vi "Get_data.vi"() -> (0 "EOF? and Error status":bool, 6 "Block Header":string)   [LabVIEW 2022 SP3]
uses:
  Controls/Block_start_and_end.ctl
  Controls/Trigger_Mode.ctl
  Globals/Meas_global.vi
  Globals/Preference_global.vi
  Globals/Trav_pos_global.vi
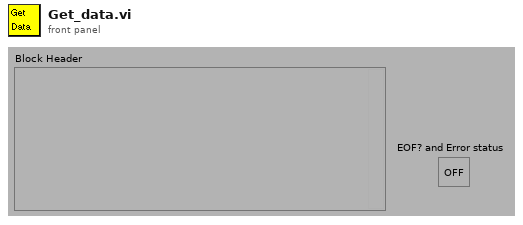
[diagram p1: front panel]
types:
  T1 = typedef "Block_start_and_end.ctl" = cluster{"Started":dbl, "Ended":dbl}
  T2 = typedef "Trigger_Mode.ctl" = enum16{"Free Running", "Start on Trigger", "Trigger Every Block", "Trigger Every Sample"}
  T3 = typedef "Post_Process.ctl" = enum16{"Take New Data", "Post Process Raw Data File"}
  T4 = typedef "PWA_Data.ctl" = enum16{"No PWA Data", "One Ch PWA"}
  T5 = typedef "Rendezvous RefNum" = refnum<k1>
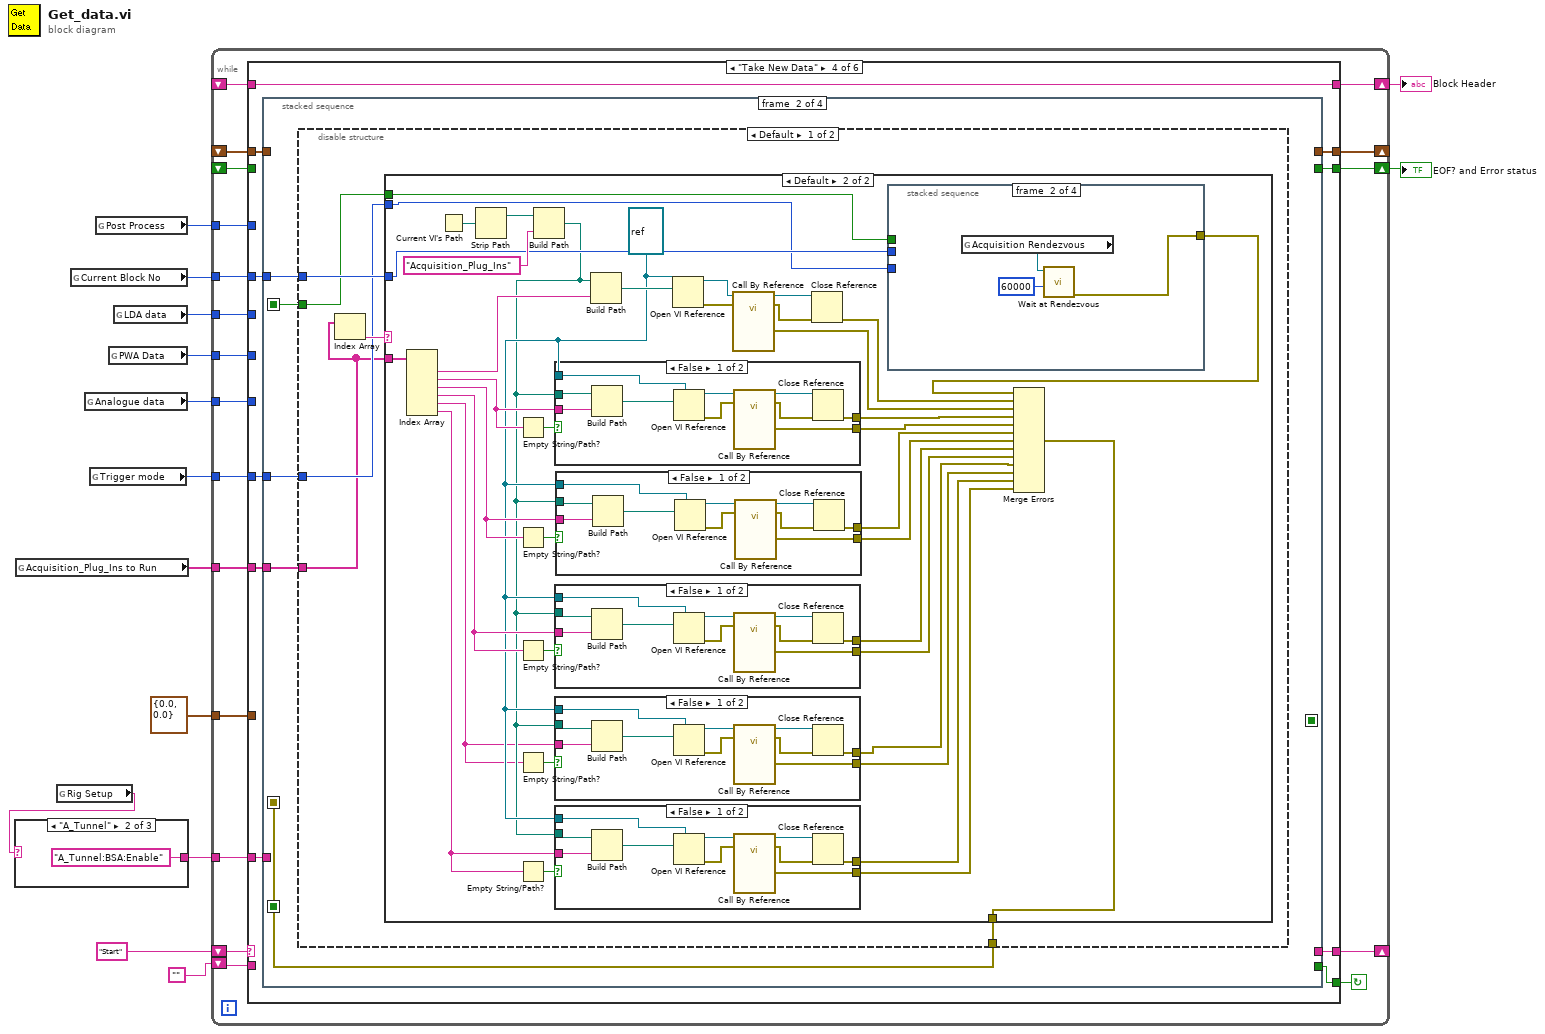
[diagram p0: block diagram]
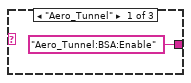
[diagram p2: hidden frame]
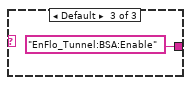
[diagram p3: hidden frame]
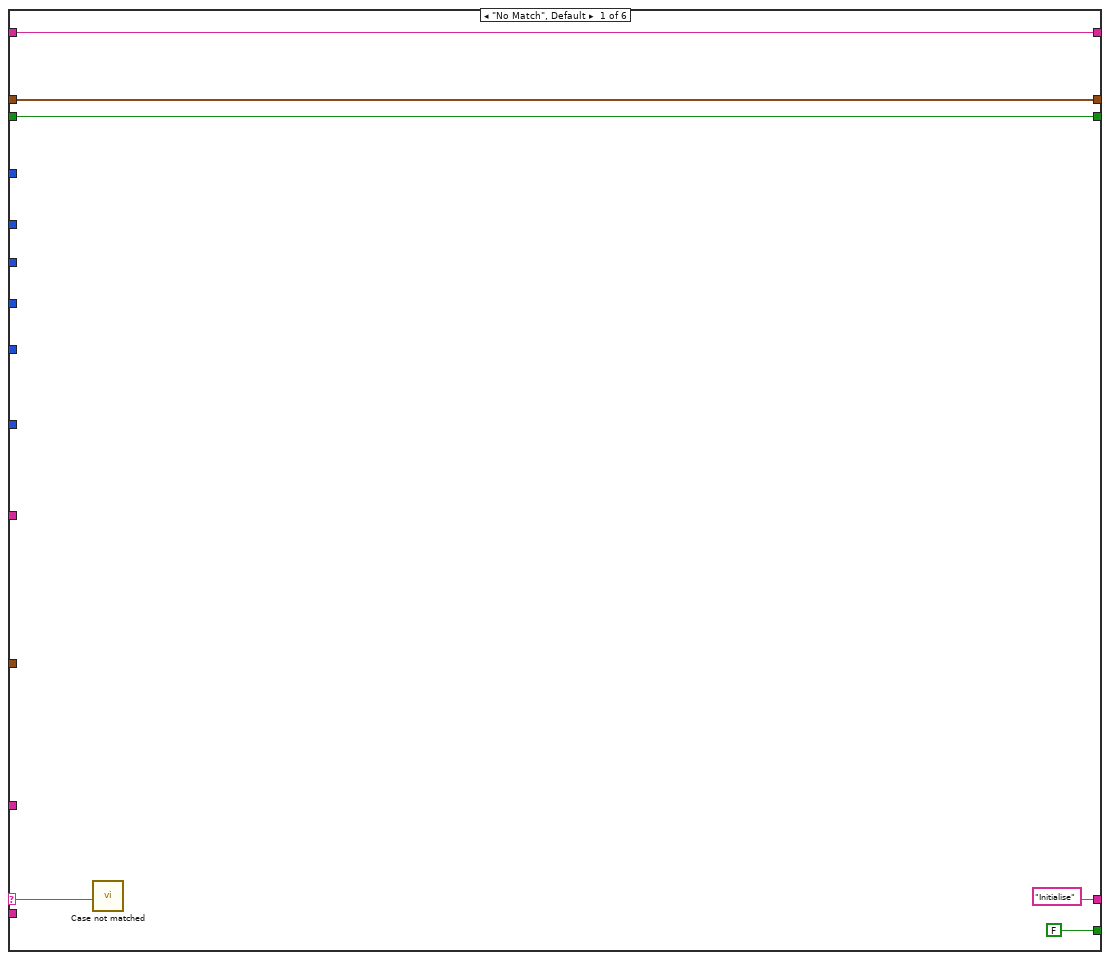
[diagram p4: hidden frame]
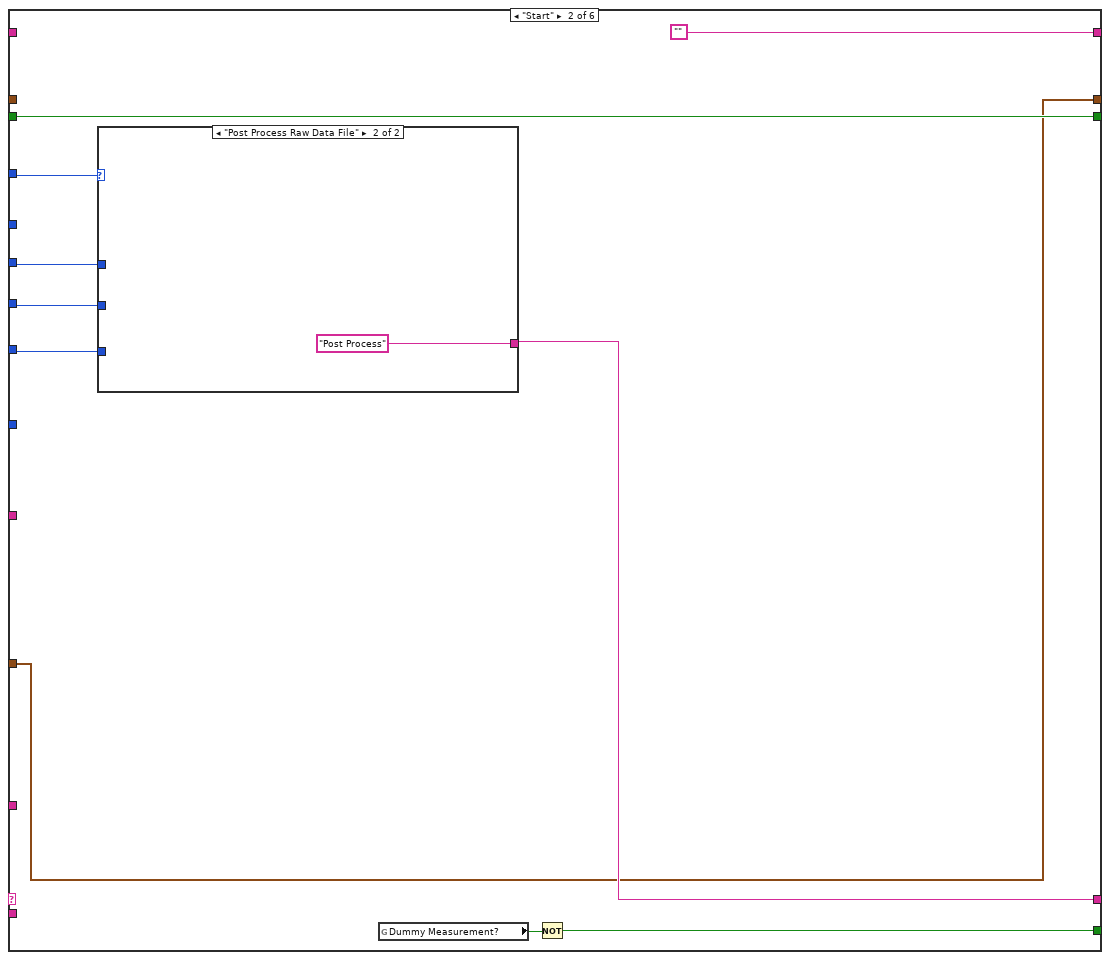
[diagram p5: hidden frame]
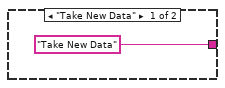
[diagram p6: hidden frame]
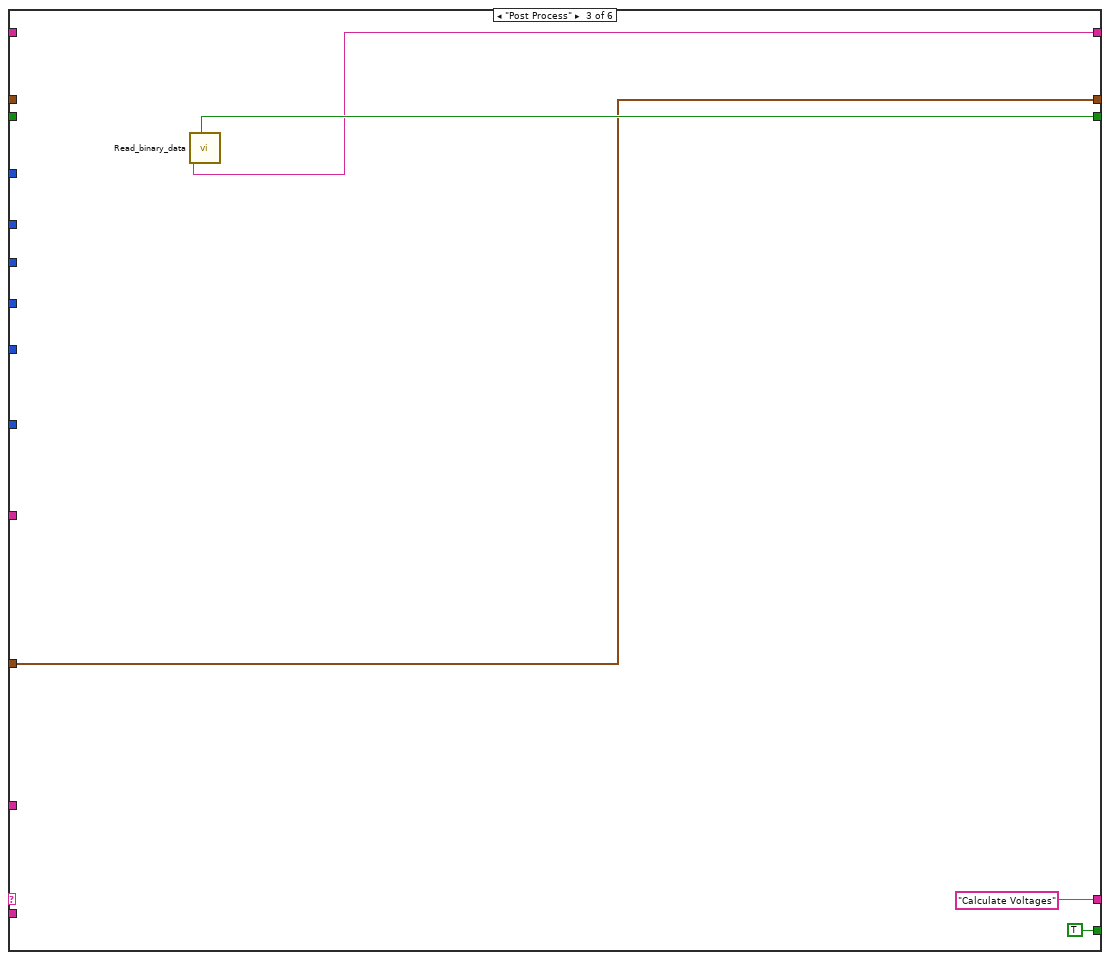
[diagram p7: hidden frame]
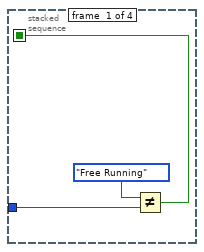
[diagram p8: hidden frame]
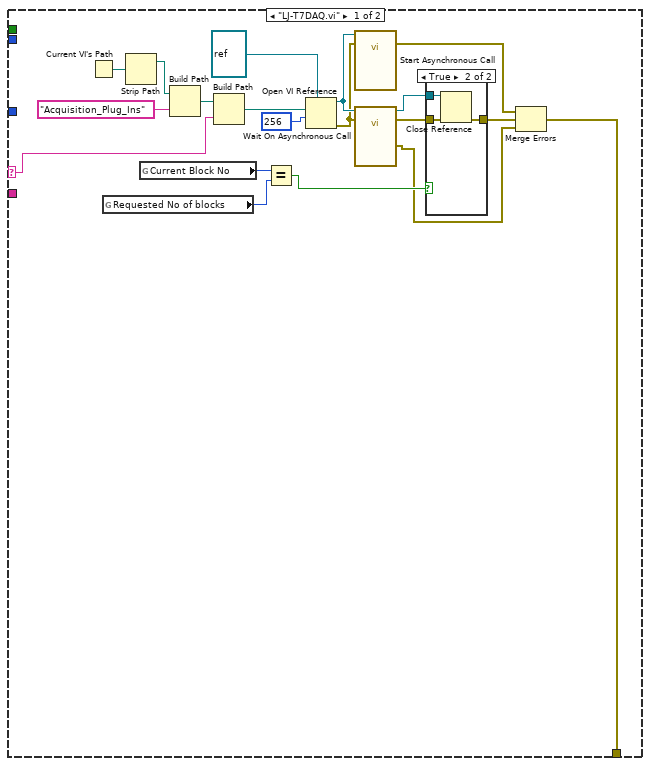
[diagram p9: hidden frame]
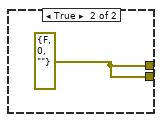
[diagram p11: hidden frame]
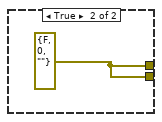
[diagram p12: hidden frame]
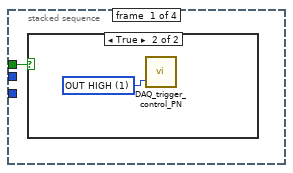
[diagram p13: hidden frame]
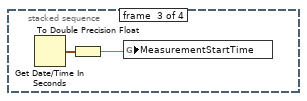
[diagram p15: hidden frame]
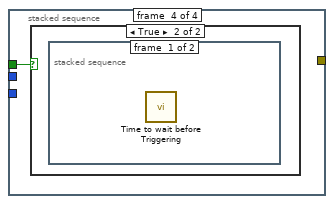
[diagram p16: hidden frame]
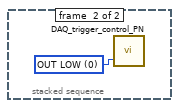
[diagram p18: hidden frame]
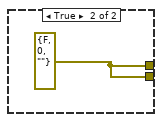
[diagram p19: hidden frame]
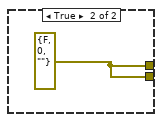
[diagram p20: hidden frame]
diagram:
  n1 = global read "Meas_global.vi" "Acquisition_Plug_Ins to Run"() -> (w1:string[])
  n2 = global read "Preference_global.vi" "Rig Setup"() -> (w2:string)
  n3 = case shown="\"A_Tunnel\"" w2 {
    tunnel: ["Aero_Tunnel:BSA:Enable" "A_Tunnel:BSA:Enable" "EnFlo_Tunnel:BSA:Enable"] -> w3
    frame "Aero_Tunnel" {
    }
    frame "A_Tunnel" {
    }
    frame Default {
    }
  }
  n4 = global read "Meas_global.vi" "Current Block No"() -> (w11:i32)
  n5 = global read "Meas_global.vi" "Analogue data"() -> (w10:enum16{"No Analogue data", "Take Analogue data"})
  n6 = global read "Meas_global.vi" "Trigger mode"() -> (w6:T2)
  n7 = global read "Meas_global.vi" "Post Process"() -> (w12:T3)
  n8 = global read "Meas_global.vi" "PWA Data"() -> (w8:T4)
  n9 = global read "Meas_global.vi" "LDA data"() -> (w9:enum16{"No LDA data", "Take LDA data"})
  n10 = while {
    shift-left: "Start" -> [w34]
    shift-right: [w35] -> _
    shift-right: [w33] -> _
    shift-left: _ -> [w32]
    shift-right: [w31] -> w14
    shift-left: _ -> [w30]
    tunnel: T1 {"Started"=0.0, "Ended"=0.0} ("Block Timings") -> [w29]
    tunnel: w12 -> [w28]
    tunnel: w11 -> [w27]
    tunnel: w10 -> [w26]
    tunnel: w9 -> [w25]
    tunnel: w8 -> [w24]
    shift-right: [w22] -> w7
    shift-left: _ -> [w23]
    tunnel: w6 -> [w21]
    shift-left: "" -> [w20]
    tunnel: w3 -> [w19]
    tunnel: w1 -> [w18]
    stop <- w36 continue-if-true
    n11 = case shown="\"Take New Data\"" w34 {
      selector: w34 -> [w37 _ _ _ _ _]
      tunnel: [FALSE w43 TRUE w65 w299 FALSE] -> w36
      tunnel: ["Initialise" w50 "Calculate Voltages" w66 "Save Raw Data" "End"] -> w35
      tunnel: [w40 w45 w55 w67 w303 w313] -> w33
      tunnel: w32 -> [w40 _ _ w68 w303 w313]
      tunnel: [w38 w52 w57 w64 w302 w314] -> w31
      tunnel: w30 -> [w38 w52 _ _ w302 w314]
      tunnel: w29 -> [_ w45 w55 _ _ _]
      tunnel: w28 -> [_ w51 _ _ _ _]
      tunnel: w27 -> [_ _ _ w62 _ w308]
      tunnel: w26 -> [_ w49 _ _ _ _]
      tunnel: w25 -> [_ w48 _ _ _ _]
      tunnel: w24 -> [_ w47 _ _ _ _]
      tunnel: [w39 "" w56 w69 w298 w310] -> w22
      tunnel: w23 -> [w39 _ _ w69 w298 w309]
      tunnel: w21 -> [_ _ _ w63 _ _]
      tunnel: w20 -> [_ _ _ _ _ _]
      tunnel: w19 -> [_ _ _ w61 _ _]
      tunnel: w18 -> [_ _ _ w60 _ _]
      frame "No Match", Default {
        n12 = call "Case not matched.vi"("Case Name not Matched"=w37) -> ()
      }
      frame "Start" {
        n13 = case shown="\"Post Process Raw Data File\"" w51 {
          tunnel: ["Take New Data" "Post Process"] -> w50
          tunnel: w49 -> [_ _]
          tunnel: w48 -> [_ _]
          tunnel: w47 -> [_ _]
          frame "Take New Data" {
          }
          frame "Post Process Raw Data File" {
          }
        }
        n14 = global read "Trav_pos_global.vi" "Dummy Measurement?"() -> (w44:bool)
        n15 = Not(x=w44) -> (.not. x?=w43:bool)
      }
      frame "Post Process" {
        n16 = call "Read_binary_data.vi"() -> ("EOF?"=w57:bool, "Block Header"=w56:string)  [unwired: 8 out]
      }
      frame "Take New Data" {
        n17 = stacked-sequence {
          seq-local: [_ w75 _ _] -> [_ _ w266 _]
          seq-local: [w70 _ _ _] -> [_ w74 _ _]
          seq-local: [_ _ w257 _] -> [_ _ _ w285]
          seq-local: [_ _ w254 _] -> [_ _ _ w282]
          tunnel: w68 -> [_ _ w274 _]
          tunnel: [_ _ w272 _] -> w67
          tunnel: [_ _ "Calculate Voltages" _] -> w66
          tunnel: [_ _ TRUE _] -> w65
          tunnel: [_ _ _ w283] -> w64
          tunnel: w63 -> [w72 w77 _ _]
          tunnel: w62 -> [_ w76 _ _]
          tunnel: w61 -> [_ _ w256 w284]
          tunnel: w60 -> [_ w73 _ _]
          frame #0 {
            n18 = Not Equal?(x=Trigger_Mode."Free Running" ("Trigger mode"), y=w72) -> (x != y?=w70:bool)
          }
          frame #1 {
            n19 = disable-structure shown="Default" {
              disable-tunnel: [w83 w212] -> w75
              disable-tunnel: w77 -> [w79 _]
              disable-tunnel: w76 -> [w81 _]
              disable-tunnel: w74 -> [w80 _]
              disable-tunnel: w73 -> [w78 w210]
              frame condition #0 (active) {
                n20 = Index Array(array=w78) -> (element=w82:string)  [unwired: 1 in]
                n21 = case shown="Default" w82 {
                  selector: w82 -> [w84 _]
                  tunnel: [w86 w129] -> w83
                  tunnel: w78 -> [_ w137]
                  tunnel: w80 -> [_ w119]
                  tunnel: w81 -> [_ w120]
                  tunnel: w79 -> [_ w118]
                  frame "LJ-T7DAQ.vi" {
                    n22 = Current VI's Path() -> (path=w99:path)
                    n23 = global read "Meas_global.vi" "Requested No of blocks"() -> (w100:i32)
                    n24 = Strip Path(path=w99) -> (stripped path=w97:path)  [unwired: 1 out]
                    n25 = global read "Meas_global.vi" "Current Block No"() -> (w101:i32)
                    n26 = Build Path(base path=w97, name or relative path="Acquisition_Plug_Ins") -> (appended path=w96:path)
                    n27 = Build Path(base path=w96, name or relative path=w84) -> (appended path=w95:path)
                    n28 = Equal?(x=w101, y=w100) -> (x = y?=w102:bool)
                    n29 = Open VI Reference(type specifier VI Refnum (for type only)=refnum<vi> refnum, vi path=w95, options=256) -> (vi reference=w93:refnum<vi>, error out=w92:errorcluster)  [unwired: 3 in]
                    n30 = call-by-ref "Start Asynchronous Call"(reference=w93, error in=w92) -> (error out=w88:errorcluster)  [unwired: 1 in, 2 out]
                    n31 = call-by-ref "Wait On Asynchronous Call"(reference=w93, error in=w92) -> (reference out=w90:refnum<vi>, error out=w89:errorcluster, 0:"error out"=w85:errorcluster)  [unwired: 1 in]
                    n32 = case shown="True" w102 {
                      tunnel: [w103 w106] -> w87
                      tunnel: w89 -> [w103 w105]
                      tunnel: w90 -> [_ w104]
                      frame False {
                      }
                      frame True {
                        n33 = Close Reference(reference=w104, error in (no error)=w105) -> (error out=w106:errorcluster)
                      }
                    }
                    n34 = Merge Errors(w88, w87, w85) -> (w86:errorcluster)
                  }
                  frame Default {
                    w115 = refnum<vi> refnum ("type specifier VI Refnum (for type only)")
                    n35 = Index Array(array=w137) -> (element #1=w136:string, element #2=w134:string, element #3=w125:string, element #4=w126:string, element #5=w113:string, element #6=w112:string)  [unwired: 6 in]
                    n36 = Current VI's Path() -> (path=w145:path)
                    n37 = Strip Path(path=w145) -> (stripped path=w143:path)  [unwired: 1 out]
                    n38 = Empty String/Path?(string/path=w134) -> (empty?=w135:bool)
                    n39 = Empty String/Path?(string/path=w125) -> (empty?=w128:bool)
                    n40 = Empty String/Path?(string/path=w126) -> (empty?=w127:bool)
                    n41 = Empty String/Path?(string/path=w113) -> (empty?=w117:bool)
                    n42 = Empty String/Path?(string/path=w112) -> (empty?=w116:bool)
                    n43 = Build Path(base path=w143, name or relative path="Acquisition_Plug_Ins") -> (appended path=w114:path)
                    n44 = case shown="False" w135 {
                      tunnel: w114 -> [w203 _]
                      tunnel: w134 -> [w202 _]
                      tunnel: w115 -> [w199 _]
                      tunnel: [w201 w209] -> w131
                      tunnel: [w200 w209] -> w130
                      frame False {
                        n45 = Build Path(base path=w203, name or relative path=w202) -> (appended path=w204:path)
                        n46 = Open VI Reference(type specifier VI Refnum (for type only)=w199, vi path=w204) -> (vi reference=w205:refnum<vi>, error out=w206:errorcluster)  [unwired: 4 in]
                        n47 = call-by-ref "?"(reference=w205, error in=w206) -> (reference out=w208:refnum<vi>, error out=w207:errorcluster, "error out"=w200:errorcluster)  [unwired: 1 in]
                        n48 = Close Reference(reference=w208, error in (no error)=w207) -> (error out=w201:errorcluster)
                      }
                      frame True {
                        w209 = errorcluster {"status"=FALSE, "code"=0, "source"=""} ("error out")
                      }
                    }
                    n49 = case shown="False" w127 {
                      tunnel: w114 -> [w181 _]
                      tunnel: w126 -> [w180 _]
                      tunnel: [w179 w187] -> w122
                      tunnel: [w178 w187] -> w121
                      tunnel: w115 -> [w177 _]
                      frame False {
                        n50 = Build Path(base path=w181, name or relative path=w180) -> (appended path=w182:path)
                        n51 = Open VI Reference(type specifier VI Refnum (for type only)=w177, vi path=w182) -> (vi reference=w183:refnum<vi>, error out=w184:errorcluster)  [unwired: 4 in]
                        n52 = call-by-ref "?"(reference=w183, error in=w184) -> (reference out=w186:refnum<vi>, error out=w185:errorcluster, "error out"=w178:errorcluster)  [unwired: 1 in]
                        n53 = Close Reference(reference=w186, error in (no error)=w185) -> (error out=w179:errorcluster)
                      }
                      frame True {
                        w187 = errorcluster {"status"=FALSE, "code"=0, "source"=""} ("error out")
                      }
                    }
                    n54 = case shown="False" w117 {
                      tunnel: w114 -> [w161 _]
                      tunnel: w113 -> [w160 _]
                      tunnel: [w159 w167] -> w111
                      tunnel: [w158 w167] -> w110
                      tunnel: w115 -> [w157 _]
                      frame False {
                        n55 = Build Path(base path=w161, name or relative path=w160) -> (appended path=w162:path)
                        n56 = Open VI Reference(type specifier VI Refnum (for type only)=w157, vi path=w162) -> (vi reference=w163:refnum<vi>, error out=w164:errorcluster)  [unwired: 4 in]
                        n57 = call-by-ref "?"(reference=w163, error in=w164) -> (reference out=w166:refnum<vi>, error out=w165:errorcluster, "error out"=w158:errorcluster)  [unwired: 1 in]
                        n58 = Close Reference(reference=w166, error in (no error)=w165) -> (error out=w159:errorcluster)
                      }
                      frame True {
                        w167 = errorcluster {"status"=FALSE, "code"=0, "source"=""} ("error out")
                      }
                    }
                    n59 = case shown="False" w116 {
                      tunnel: w114 -> [w150 _]
                      tunnel: w112 -> [w149 _]
                      tunnel: [w148 w156] -> w109
                      tunnel: [w147 w156] -> w108
                      tunnel: w115 -> [w146 _]
                      frame False {
                        n60 = Build Path(base path=w150, name or relative path=w149) -> (appended path=w151:path)
                        n61 = Open VI Reference(type specifier VI Refnum (for type only)=w146, vi path=w151) -> (vi reference=w152:refnum<vi>, error out=w153:errorcluster)  [unwired: 4 in]
                        n62 = call-by-ref "?"(reference=w152, error in=w153) -> (reference out=w155:refnum<vi>, error out=w154:errorcluster, "error out"=w147:errorcluster)  [unwired: 1 in]
                        n63 = Close Reference(reference=w155, error in (no error)=w154) -> (error out=w148:errorcluster)
                      }
                      frame True {
                        w156 = errorcluster {"status"=FALSE, "code"=0, "source"=""} ("error out")
                      }
                    }
                    n64 = case shown="False" w128 {
                      tunnel: w114 -> [w192 _]
                      tunnel: w125 -> [w191 _]
                      tunnel: [w190 w198] -> w124
                      tunnel: [w189 w198] -> w123
                      tunnel: w115 -> [w188 _]
                      frame False {
                        n65 = Build Path(base path=w192, name or relative path=w191) -> (appended path=w193:path)
                        n66 = Open VI Reference(type specifier VI Refnum (for type only)=w188, vi path=w193) -> (vi reference=w194:refnum<vi>, error out=w195:errorcluster)  [unwired: 4 in]
                        n67 = call-by-ref "?"(reference=w194, error in=w195) -> (reference out=w197:refnum<vi>, error out=w196:errorcluster, "error out"=w189:errorcluster)  [unwired: 1 in]
                        n68 = Close Reference(reference=w197, error in (no error)=w196) -> (error out=w190:errorcluster)
                      }
                      frame True {
                        w198 = errorcluster {"status"=FALSE, "code"=0, "source"=""} ("error out")
                      }
                    }
                    n69 = Build Path(base path=w114, name or relative path=w136) -> (appended path=w142:path)
                    n70 = Open VI Reference(type specifier VI Refnum (for type only)=w115, vi path=w142) -> (vi reference=w141:refnum<vi>, error out=w140:errorcluster)  [unwired: 4 in]
                    n71 = call-by-ref "?"(reference=w141, error in=w140) -> (reference out=w138:refnum<vi>, error out=w139:errorcluster, "error out"=w132:errorcluster)  [unwired: 1 in]
                    n72 = Close Reference(reference=w138, error in (no error)=w139) -> (error out=w133:errorcluster)
                    n73 = stacked-sequence {
                      tunnel: [_ w172 _ _] -> w107
                      tunnel: w119 -> [w168 _ _ w175]
                      tunnel: w120 -> [_ _ _ _]
                      tunnel: w118 -> [_ _ _ _]
                      frame #0 {
                        n74 = case shown="True" w168 {
                          frame False {
                          }
                          frame True {
                            w169 = u8 1 items=["OUT LOW", "OUT HIGH", "IN READ"] ("Action")
                            n75 = call "DAQ_trigger_control_PN.vi"("Action"=w169) -> ()  [unwired: 1 in, 3 out]
                          }
                        }
                      }
                      frame #1 {
                        n76 = global read "Meas_global.vi" "Acquisition Rendezvous"() -> (w171:T5)
                        n77 = call <vilib>:"Wait at Rendezvous.vi"("ms timeout (-1)"=60000, "rendezvous"=w171) -> ("error out"=w172:errorcluster)  [unwired: 3 in, 2 out]
                      }
                      frame #2 {
                        n78 = Get Date/Time In Seconds() -> (seconds since 1Jan1904=w174:timestamp)
                        n79 = To Double Precision Float(number=w174) -> (double precision float=w173:dbl)
                        n80 = global write "Meas_global.vi" "MeasurementStartTime"(w173) -> ()
                      }
                      frame #3 {
                        n81 = case shown="True" w175 {
                          frame False {
                          }
                          frame True {
                            n82 = stacked-sequence {
                              frame #0 {
                                n83 = call "Time to wait before Triggering.vi"() -> ()  [unwired: 12 in]
                              }
                              frame #1 {
                                w176 = u8 0 items=["OUT LOW", "OUT HIGH", "IN READ"] ("Action")
                                n84 = call "DAQ_trigger_control_PN.vi"("Action"=w176) -> ()  [unwired: 1 in, 3 out]
                              }
                            }
                          }
                        }
                      }
                    }
                    n85 = Merge Errors(w107, w133, w132, w131, w130, w124, w123, w122, w121, w111, w110, w109, w108) -> (w129:errorcluster)
                  }
                }
              }
              frame condition #1 {
                # "Experimenting with full DAQmx on Mac..."
                n86 = Index Array(array=w210) -> (element=w211:string)  [unwired: 1 in]
                n87 = case shown="\"False\", Default" w211 {
                  selector: w211 -> [_ w220 w239]
                  tunnel: [errorcluster {"status"=TRUE, "code"=0, "source"=""} ("Error Out") w221 w240] -> w212
                  frame "False", Default {
                    n88 = One Button Dialog(message="Sorry; that DAQ plugin is not currently supported on the Mac...", button name ("OK")="Bugger!") -> (true=w214:bool)
                    n89 = Stop(stop? (T)=w214) -> ()
                  }
                  frame "LJ-T7DAQ.vi" {
                    n90 = Current VI's Path() -> (path=w222:path)
                    n91 = global read "Meas_global.vi" "Requested No of blocks"() -> (w219:i32)
                    n92 = Strip Path(path=w222) -> (stripped path=w224:path)  [unwired: 1 out]
                    n93 = global read "Meas_global.vi" "Current Block No"() -> (w218:i32)
                    n94 = Build Path(base path=w224, name or relative path="Acquisition_Plug_Ins") -> (appended path=w225:path)
                    n95 = Build Path(base path=w225, name or relative path=w220) -> (appended path=w226:path)
                    n96 = Equal?(x=w218, y=w219) -> (x = y?=w217:bool)
                    n97 = Open VI Reference(type specifier VI Refnum (for type only)=refnum<vi> refnum, vi path=w226, options=256) -> (vi reference=w228:refnum<vi>, error out=w229:errorcluster)  [unwired: 3 in]
                    n98 = call-by-ref "Start Asynchronous Call"(reference=w228, error in=w229) -> (error out=w233:errorcluster)  [unwired: 1 in, 2 out]
                    n99 = call-by-ref "Wait On Asynchronous Call"(reference=w228, error in=w229) -> (reference out=w231:refnum<vi>, error out=w232:errorcluster)  [unwired: 1 in, 1 out]
                    n100 = case shown="True" w217 {
                      tunnel: [w235 w238] -> w234
                      tunnel: w232 -> [w235 w237]
                      tunnel: w231 -> [_ w236]
                      frame False {
                      }
                      frame True {
                        n101 = Close Reference(reference=w236, error in (no error)=w237) -> (error out=w238:errorcluster)
                      }
                    }
                    n102 = Merge Errors(w233, w234) -> (w221:errorcluster)
                  }
                  frame "ADAM_Server_Channels.vi", "NI-DAQmx.vi", "Simulate_kernal.vi" {
                    n103 = Current VI's Path() -> (path=w241:path)
                    n104 = Strip Path(path=w241) -> (stripped path=w243:path)  [unwired: 1 out]
                    n105 = Build Path(base path=w243, name or relative path="Acquisition_Plug_Ins") -> (appended path=w244:path)
                    n106 = Build Path(base path=w244, name or relative path=w239) -> (appended path=w245:path)
                    n107 = Open VI Reference(type specifier VI Refnum (for type only)=refnum<vi> refnum, vi path=w245, options=256) -> (vi reference=w247:refnum<vi>, error out=w248:errorcluster)  [unwired: 3 in]
                    n108 = call-by-ref "Wait On Asynchronous Call"(reference=w247, error in=w248) -> (reference out=w250:refnum<vi>, error out=w251:errorcluster)  [unwired: 1 in, 1 out]
                    n109 = call-by-ref "Start Asynchronous Call"(reference=w247, error in=w248) -> (error out=w252:errorcluster)  [unwired: 1 in, 2 out]
                    n110 = Close Reference(reference=w250, error in (no error)=w251) -> (error out=w253:errorcluster)
                    n111 = Merge Errors(w252, w253) -> (w240:errorcluster)
                  }
                }
              }
            }
          }
          frame #2 {
            n112 = Get Date/Time In Seconds() -> (seconds since 1Jan1904=w275:timestamp)
            n113 = global read "Meas_global.vi" "Acquisition Rendezvous"() -> (w267:T5)
            n114 = To Double Precision Float(number=w275) -> (double precision float=w273:dbl)
            n115 = call <vilib>:"Destroy Rendezvous.vi"("rendezvous"=w267) -> ("error out"=w264:errorcluster)  [unwired: 5 in, 1 out]
            n116 = global read "Meas_global.vi" "MeasurementStartTime"() -> (w255:dbl)
            n117 = Merge Errors(w264, w266) -> (w265:errorcluster)
            n118 = Bundle By Name(cluster=w274, "Started"=w255, "Ended"=w273) -> (w272:T1)
            n119 = Unbundle By Name(w265) -> ("status"=w254:bool, "source"=w262:string)
            n120 = call "EnFlo_Error_Handler.vi"("error in (no error)"=w265, "Error Type"="Acquisition_Vi", "Dialog Box (F)"=FALSE ("Dialog Box (T)")) -> ()  [unwired: 3 out]
            n121 = global write "Meas_global.vi" "Acquisition Complete?"(TRUE ("Acquisition Complete?")) -> ()
            n122 = Match Pattern(string=w262, regular expression="no answer from BSA Processor") -> (offset past match=w260:i32)  [unwired: 1 in, 3 out]
            n123 = Greater Than 0?(x=w260) -> (x > 0?=w259:bool)
            n124 = Compound Arithmetic op=AND(w254, w259) -> (w258:bool)
            n125 = case shown="True" w258 {
              tunnel: [FALSE w278] -> w257
              tunnel: w256 -> [_ w277]
              frame False {
              }
              frame True {
                n126 = call "Get_Current_Scan_client.vi"("singleChannel"=w277) -> ("Numerical Values"=w281:dbl[])  [unwired: 1 in, 3 out]
                n127 = Index Array(array=w281) -> (element=w280:dbl)  [unwired: 1 in]
                n128 = Greater?(x=w280, y=0.5) -> (0:w278:bool)
              }
            }
          }
          frame #3 {
            n129 = case shown="True" w285 {
              tunnel: w284 -> [_ w289]
              tunnel: [w286 TRUE] -> w283
              tunnel: w282 -> [w286 _]
              frame False {
              }
              frame True {
                # "Routine to Restart F60 BSA"
                n130 = Build Array(w289) -> (w288:string[])
                n131 = stacked-sequence {
                  tunnel: w288 -> [w291 _ w295 _]
                  frame #0 {
                    n132 = call "ASYNC_Adam_client.vi"("Values"=dbl[] [0.0], "Channel Names"=w291) -> ()  [unwired: 1 in, 2 out]
                  }
                  frame #1 {
                    n133 = call "Wait_Seconds_with_display_Simple.vi"("Message"="Waiting for BSA to turn off", "Seconds to wait"=20.0) -> ()  [unwired: 1 in, 1 out]
                  }
                  frame #2 {
                    n134 = call "ASYNC_Adam_client.vi"("Values"=dbl[] [1.0], "Channel Names"=w295) -> ()  [unwired: 1 in, 2 out]
                  }
                  frame #3 {
                    n135 = call "Wait_Seconds_with_display_Simple.vi"("Message"="Waiting for BSA to start up", "Seconds to wait"=180.0) -> ()  [unwired: 1 in, 1 out]
                  }
                }
              }
            }
          }
        }
      }
      frame "Calculate Voltages" {
        n136 = global read "Meas_global.vi" "Raw data option"() -> (w301:enum16{"Save raw data", "Raw data not saved"})
        n137 = case shown="\"Raw data not saved\"" w301 {
          tunnel: [TRUE FALSE] -> w299
          frame "Save raw data" {
          }
          frame "Raw data not saved" {
          }
        }
      }
      frame "Save Raw Data" {
        n138 = Greater?(x=w308, y=1) -> (0:w306:bool)
        n139 = call "Save_Raw_data.vi"("Add to Block Header"=w309, "append to file? (new file:F)"=w306, "Block Timings"=w313) -> ("Block Header"=w310:string)  [unwired: 6 in]
      }
    }
  }
  "EOF? and Error status" <- w14
  "Block Header" <- w7
